vi "Flip Image.vi"   [LabVIEW 2020, in "g_ar_toolkit.image.lvlib"]
doc: "Resize the image source into the destination.\n\nMore information on the interpolation mode can be found at https://docs.opencv.org/4.8.0/da/d54/group__imgproc__transform.html#ga5bb5a1fea74ea38e1a5445ca803ff121"
uses:
  g_ar_toolkit.image.lvlib
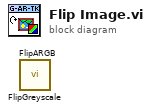
[diagram p0: block diagram]
diagram:
  n1 = call "FlipGreyscale.vi"() -> ()  [unwired: 10 in, 2 out]
  n2 = call "FlipARGB.vi"() -> ()  [unwired: 10 in, 2 out]
